vi "PRAT DO1.vi"(0 "VISA session":refnum<visa-resource-name>="MW100", 5 "PRAT Channels":T2, 7 "Normally Open Valve":T1, 11 "Error In":errorcluster) -> (4 "dup VISA session":refnum<visa-resource-name>, 15 "error out":errorcluster)   [LabVIEW 2016]
uses:
  Type Definitions/PRAT Channel Settings.ctl
  Type Definitions/HEWH Normally Open Valve Control.ctl
panel:
  # "PWR_MAIN: CLOSED = POWER OFF"
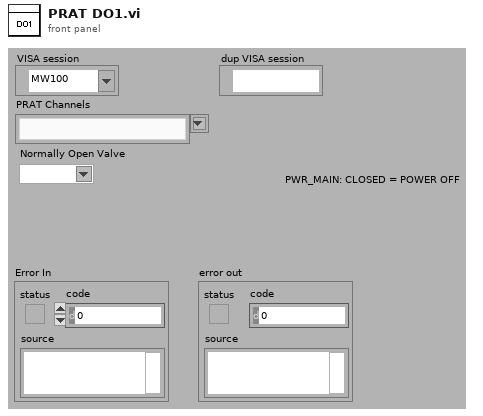
[diagram p1: front panel]
types:
  T1 = typedef "HEWH Normally Open Valve Control.ctl" = string
  T2 = typedef "PRAT Channel Settings.ctl" = string
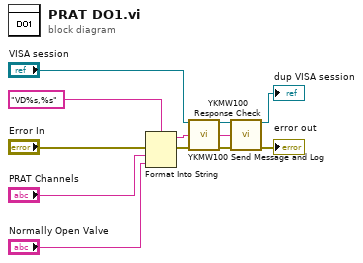
[diagram p0: block diagram]
diagram:
  n1 = Format Into String(format string="VD%s,%s", error in="Error In", "PRAT Channels", "Normally Open Valve") -> (resulting string=w8:string, error out=w9:errorcluster)  [unwired: 1 in]
  n2 = call "YKMW100 Send Message and Log.vi"("VISA session"="VISA session", "Send Message (\"\")"=w8, "error in (no error)"=w9) -> ("dup VISA session"=w7:refnum<visa-resource-name>, "Read Buffer"=w5:string, "error out"=w6:errorcluster)  [unwired: 10 in]
  n3 = call "YKMW100 Response Check.vi"("VISA session"=w7, "Message In (\"\")"=w5, "error in (no error)"=w6) -> ("dup VISA session"=→"dup VISA session":refnum<visa-resource-name>, "error out"=→"error out":errorcluster)  [unwired: 8 in, 3 out]
